vi "LaserInitilisation.vi"(0 "WaveformGraph in":refnum<vi>, 1 "Knob Refnum 2":refnum<vi>, 2 "DigNum Refnum":refnum<vi>, 3 "Knob Refnum 3":refnum<vi>, 4 "Knob Refnum 4":refnum<vi>, 5 "error in (no error)":errorcluster, 6 "Bool Refnum 2":refnum<vi>, 7 "reference":refnum<vi>, 8 "WFGraph Refnum in":refnum<vi>, 10 "Knob Refnum":refnum<vi>, 11 "Bool Refnum":refnum<vi>) -> (19 "error out":errorcluster)   [LabVIEW 2011]
uses:
  Variables/GlobalLaserInterface.vi
  Variables/GlobalLaserOnOff.vi
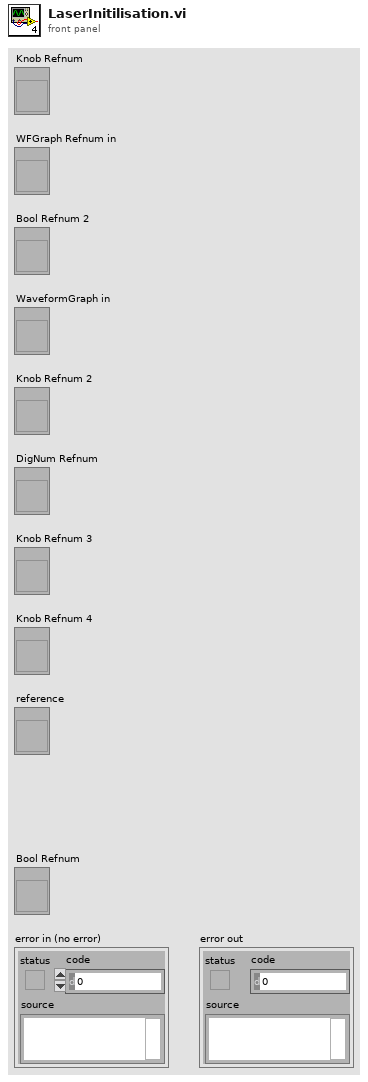
[diagram p1: front panel]
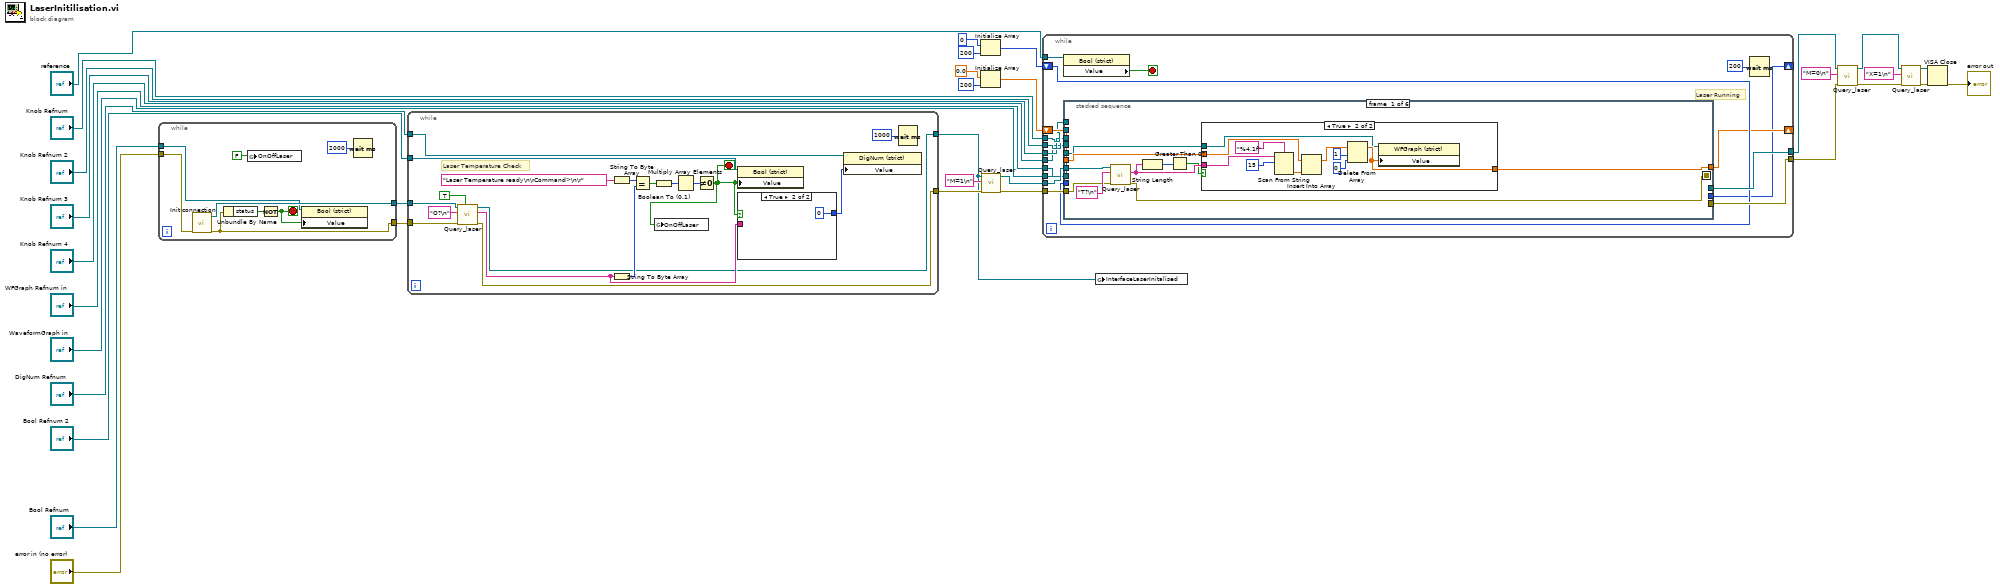
[diagram p0: block diagram]
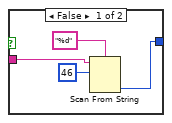
[diagram p2: hidden frame]
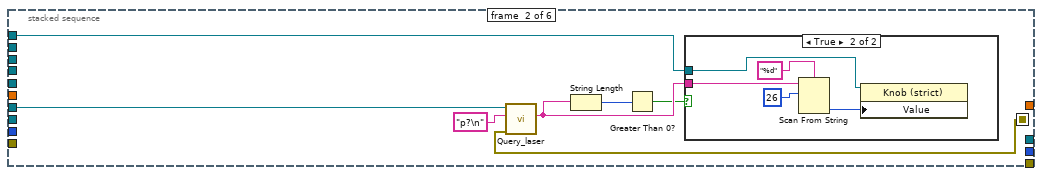
[diagram p4: hidden frame]
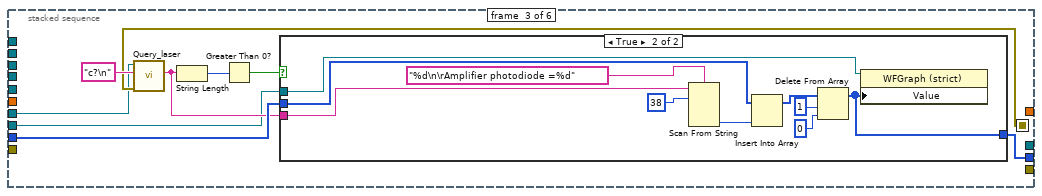
[diagram p6: hidden frame]
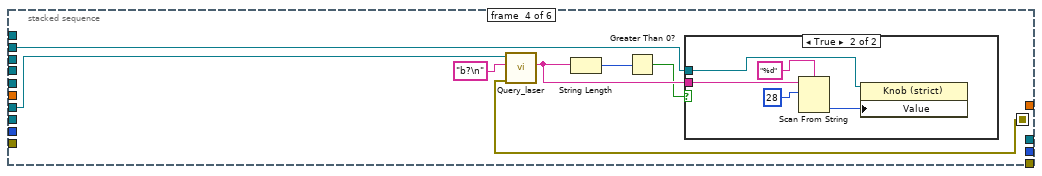
[diagram p8: hidden frame]
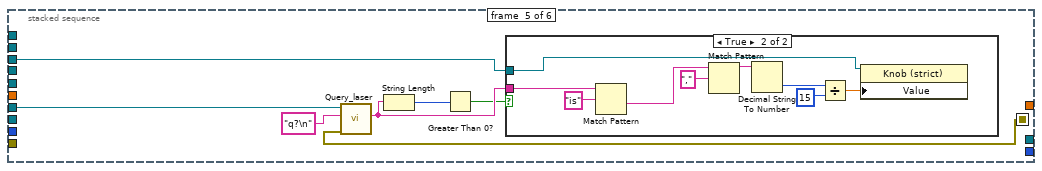
[diagram p10: hidden frame]
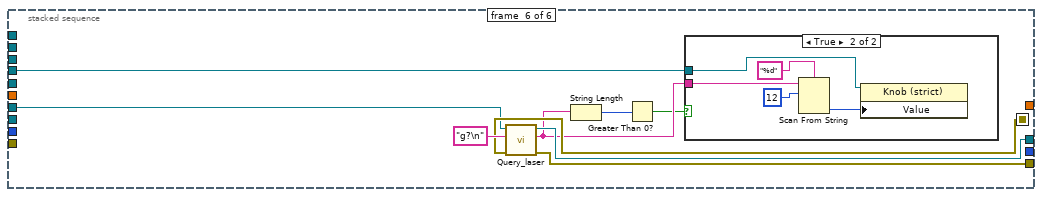
[diagram p12: hidden frame]
diagram:
  n1 = while {
    tunnel: [w39] -> w18
    tunnel: [w38] -> w19
    tunnel: "error in (no error)" -> [w37]
    tunnel: "Bool Refnum" -> [w35]
    stop <- w36 stop-if-true
    n2 = call "Init connection.vi"("error in"=w37) -> ("error constant"=w39:errorcluster, "VISA resource name 2"=w38:refnum<visa-resource-name>)  [unwired: 9 in]
    n3 = Unbundle By Name(w39) -> ("status"=w40:bool)
    n4 = global write "GlobalLaserOnOff.vi" "OnOffLaser"(FALSE ("OnOffLaser")) -> ()
    n5 = Not(x=w40) -> (.not. x?=w36:bool)
    n6 = property on="Property Node" class="Bool (strict)"(reference=w35, "Value"=w36) -> ()  [unwired: 1 in, 2 out]
    n7 = Wait (ms)(milliseconds to wait=2000) -> ()  [unwired: 1 out]
  }
  n8 = while {
    tunnel: w19 -> [w57]
    tunnel: w18 -> [w56]
    tunnel: [w47] -> w1
    tunnel: [w49] -> w21
    tunnel: "DigNum Refnum" -> [w44]
    tunnel: "Bool Refnum 2" -> [w43]
    stop <- w42 stop-if-true
    # "Laser Temperature Check"
    n9 = call "Query_laser.vi"("Reset?"=TRUE, "error in (no error)"=w56, "String in"="O?\n", "VISA resource name"=w57) -> ("error out"=w49:errorcluster, "String out"=w48:string, "VISA resource name 2"=w47:refnum<visa-resource-name>)  [unwired: 3 in, 1 out]
    n10 = String To Byte Array(string="Laser Temperature ready\n\rCommand>\n\r") -> (unsigned byte array=w54:u8[])
    n11 = String To Byte Array(string=w48) -> (unsigned byte array=w53:u8[])
    n12 = Equal?(x=w54, y=w53) -> (x = y?=w52:bool[])
    n13 = Boolean To (0,1)(Boolean=w52) -> (0, 1=w51:i16[])
    n14 = Multiply Array Elements(1:w51) -> (0:w50:i16)
    n15 = Not Equal To 0?(x=w50) -> (x != 0?=w42:bool)
    n16 = global write "GlobalLaserOnOff.vi" "OnOffLaser"(w42) -> ()
    n17 = property on="Property Node" class="Bool (strict)"(reference=w43, "Value"=w42) -> ()  [unwired: 1 in, 2 out]
    n18 = case shown="True" w42 {
      tunnel: w48 -> [w63 _]
      tunnel: [w61 0] -> w45
      frame False {
        n19 = Scan From String(format string="%d", input string=w63, initial scan location=46) -> (output 1=w61:i32)  [unwired: 2 in, 3 out]
      }
      frame True {
      }
    }
    n20 = property on="Property Node" class="DigNum (strict)"(reference=w44, "Value"=w45) -> ()  [unwired: 1 in, 2 out]
    n21 = Wait (ms)(milliseconds to wait=1000) -> ()  [unwired: 1 out]
  }
  n22 = Initialize Array(0, 200) -> (w4:i32[])
  n23 = Initialize Array(0.0, 200) -> (w7:dbl[])
  n24 = call "Query_laser.vi"("error in (no error)"=w21, "String in"="M=1\n", "VISA resource name"=w1) -> ("error out"=w3:errorcluster, "VISA resource name 2"=w2:refnum<visa-resource-name>)  [unwired: 4 in, 2 out]
  n25 = while {
    tunnel: w2 -> [w80]
    tunnel: w3 -> [w81]
    tunnel: [w78] -> w11
    tunnel: [w79] -> w10
    shift-right: [w74] -> _
    shift-left: w7 -> [w76]
    shift-right: [w73] -> _
    shift-left: w4 -> [w75]
    tunnel: "WaveformGraph in" -> [w71]
    tunnel: "Knob Refnum" -> [w70]
    tunnel: "WFGraph Refnum in" -> [w69]
    tunnel: "Knob Refnum 2" -> [w68]
    tunnel: "Knob Refnum 3" -> [w67]
    tunnel: "Knob Refnum 4" -> [w66]
    tunnel: "reference" -> [w65]
    stop <- w72 stop-if-true
    # "Laser Running"
    n26 = property class="Bool (strict)"(reference=w65) -> ("Value"=w72:bool)  [unwired: 1 in, 2 out]
    n27 = stacked-sequence {
      seq-local: [w86 _ _ _ _ _] -> [_ w104 w122 w140 w152 w170]
      tunnel: w80 -> [w89 w108 w119 w139 w151 w167]
      tunnel: w81 -> [w90 _ _ _ _ _]
      tunnel: [_ _ _ _ _ w169] -> w79
      tunnel: [_ _ _ _ _ w168] -> w78
      tunnel: w76 -> [w88 _ _ _ _ _]
      tunnel: w75 -> [_ _ w121 _ _ _]
      tunnel: [w87 _ _ _ _ _] -> w74
      tunnel: [_ _ w120 _ _ _] -> w73
      tunnel: w71 -> [w82 _ _ _ _ _]
      tunnel: w70 -> [_ w103 _ _ _ _]
      tunnel: w69 -> [_ _ w115 _ _ _]
      tunnel: w68 -> [_ _ _ w135 _ _]
      tunnel: w67 -> [_ _ _ _ w147 _]
      tunnel: w66 -> [_ _ _ _ _ w163]
      frame #0 {
        n28 = call "Query_laser.vi"("error in (no error)"=w90, "String in"="T?\n", "VISA resource name"=w89) -> ("error out"=w86:errorcluster, "String out"=w84:string)  [unwired: 4 in, 2 out]
        n29 = String Length(string=w84) -> (length=w85:i32)
        n30 = Greater Than 0?(x=w85) -> (x > 0?=w83:bool)
        n31 = case shown="True" w83 {
          tunnel: w88 -> [w92 w99]
          tunnel: [w92 w94] -> w87
          tunnel: w84 -> [_ w95]
          tunnel: w82 -> [_ w93]
          frame False {
          }
          frame True {
            n32 = Scan From String(format string="%4.1f", input string=w95, initial scan location=15) -> (output 1=w100:dbl)  [unwired: 2 in, 3 out]
            n33 = Insert Into Array(array=w99, new element=w100) -> (w98:dbl[])  [unwired: 1 in]
            n34 = Delete From Array(array=w98, length=1, index=0) -> (array with subset deleted=w94:dbl[])  [unwired: 1 out]
            n35 = property on="Property Node" class="WFGraph (strict)"(reference=w93, "Value"=w94) -> ()  [unwired: 1 in, 2 out]
          }
        }
      }
      frame #1 {
        n36 = call "Query_laser.vi"("error in (no error)"=w104, "String in"="p?\n", "VISA resource name"=w108) -> ("String out"=w107:string)  [unwired: 4 in, 3 out]
        n37 = String Length(string=w107) -> (length=w106:i32)
        n38 = Greater Than 0?(x=w106) -> (x > 0?=w105:bool)
        n39 = case shown="True" w105 {
          tunnel: w107 -> [_ w112]
          tunnel: w103 -> [_ w110]
          frame False {
          }
          frame True {
            n40 = Scan From String(format string="%d", input string=w112, initial scan location=26) -> (output 1=w111:i32)  [unwired: 2 in, 3 out]
            n41 = property on="Property Node" class="Knob (strict)"(reference=w110, "Value"=w111) -> ()  [unwired: 1 in, 2 out]
          }
        }
      }
      frame #2 {
        n42 = call "Query_laser.vi"("error in (no error)"=w122, "String in"="c?\n", "VISA resource name"=w119) -> ("String out"=w116:string)  [unwired: 4 in, 3 out]
        n43 = String Length(string=w116) -> (length=w118:i32)
        n44 = Greater Than 0?(x=w118) -> (x > 0?=w117:bool)
        n45 = case shown="True" w117 {
          tunnel: w121 -> [w124 w128]
          tunnel: [w124 w126] -> w120
          tunnel: w116 -> [_ w127]
          tunnel: w115 -> [_ w125]
          frame False {
          }
          frame True {
            n46 = Scan From String(format string="%d\n\rAmplifier photodiode =%d", input string=w127, initial scan location=38) -> (output 2=w129:i32)  [unwired: 4 in, 3 out]
            n47 = Insert Into Array(array=w128, new element=w129) -> (w132:i32[])  [unwired: 1 in]
            n48 = Delete From Array(array=w132, length=1, index=0) -> (array with subset deleted=w126:i32[])  [unwired: 1 out]
            n49 = property on="Property Node" class="WFGraph (strict)"(reference=w125, "Value"=w126) -> ()  [unwired: 1 in, 2 out]
          }
        }
      }
      frame #3 {
        n50 = call "Query_laser.vi"("error in (no error)"=w140, "String in"="b?\n", "VISA resource name"=w139) -> ("String out"=w137:string)  [unwired: 4 in, 3 out]
        n51 = String Length(string=w137) -> (length=w138:i32)
        n52 = Greater Than 0?(x=w138) -> (x > 0?=w136:bool)
        n53 = case shown="True" w136 {
          tunnel: w137 -> [_ w144]
          tunnel: w135 -> [_ w142]
          frame False {
          }
          frame True {
            n54 = Scan From String(format string="%d", input string=w144, initial scan location=28) -> (output 1=w143:i32)  [unwired: 2 in, 3 out]
            n55 = property on="Property Node" class="Knob (strict)"(reference=w142, "Value"=w143) -> ()  [unwired: 1 in, 2 out]
          }
        }
      }
      frame #4 {
        n56 = call "Query_laser.vi"("error in (no error)"=w152, "String in"="q?\n", "VISA resource name"=w151) -> ("String out"=w149:string)  [unwired: 4 in, 3 out]
        n57 = String Length(string=w149) -> (length=w150:i32)
        n58 = Greater Than 0?(x=w150) -> (x > 0?=w148:bool)
        n59 = case shown="True" w148 {
          tunnel: w149 -> [_ w159]
          tunnel: w147 -> [_ w160]
          frame False {
          }
          frame True {
            n60 = Match Pattern(string=w159, regular expression="is") -> (after substring=w158:string)  [unwired: 1 in, 3 out]
            n61 = Match Pattern(string=w158, regular expression=",") -> (before substring=w155:string)  [unwired: 1 in, 3 out]
            n62 = Decimal String To Number(string=w155) -> (number=w154:i32)  [unwired: 2 in, 1 out]
            n63 = Divide(x=w154, y=15) -> (x/y=w161:dbl)
            n64 = property on="Property Node" class="Knob (strict)"(reference=w160, "Value"=w161) -> ()  [unwired: 1 in, 2 out]
          }
        }
      }
      frame #5 {
        n65 = call "Query_laser.vi"("error in (no error)"=w170, "String in"="g?\n", "VISA resource name"=w167) -> ("error out"=w168:errorcluster, "String out"=w165:string, "VISA resource name 2"=w169:refnum<visa-resource-name>)  [unwired: 4 in, 1 out]
        n66 = String Length(string=w165) -> (length=w166:i32)
        n67 = Greater Than 0?(x=w166) -> (x > 0?=w164:bool)
        n68 = case shown="True" w164 {
          tunnel: w165 -> [_ w174]
          tunnel: w163 -> [_ w172]
          frame False {
          }
          frame True {
            n69 = Scan From String(format string="%d", input string=w174, initial scan location=12) -> (output 1=w173:i32)  [unwired: 2 in, 3 out]
            n70 = property on="Property Node" class="Knob (strict)"(reference=w172, "Value"=w173) -> ()  [unwired: 1 in, 2 out]
          }
        }
      }
    }
    n71 = Wait (ms)(milliseconds to wait=u32 200) -> ()  [unwired: 1 out]
  }
  n72 = global write "GlobalLaserInterface.vi" "InterfaceLaserInitalised"(w1) -> ()
  n73 = call "Query_laser.vi"("error in (no error)"=w11, "String in"="M=0\n", "VISA resource name"=w10) -> ("error out"=w12:errorcluster, "VISA resource name 2"=w13:refnum<visa-resource-name>)  [unwired: 4 in, 2 out]
  n74 = call "Query_laser.vi"("error in (no error)"=w12, "String in"="X=1\n", "VISA resource name"=w13) -> ("error out"=w16:errorcluster, "VISA resource name 2"=w15:refnum<visa-resource-name>)  [unwired: 4 in, 2 out]
  n75 = VISA Close(VISA resource name=w15, error in (no error)=w16) -> (error out=→"error out":errorcluster)
